vi "Telecommunications Parametric Testing.vi"() -> ()   [LabVIEW 2018]
doc: "The T1 Parametric testing application performs parametric testing of T1 signals. The T1 signal is a 1.544 Mb/s pulsed digital signal formed by multiplexing 24 voice channels. Each channel is sampled at 8000 samples/sec. Each sample is then converted to 8 bits using Pulse Coded Multiplexing. The 24 channels are then time-division multiplexed. Each frame, which corresponds to one sampling period, contains 192 bits ( 8 times 24) plus one bit for frame synchronization. Since frames occur at 8000 times per second, the bit rate is 1.544 Mb/s\n\nThis application performs the following parametric tests on T1 signals:\n\n1. Mask Test: Compares T1 signals with standard masks. The type of masks that are supported are ITU G.703 mask, EIA/TIA 547 and ANSI T1.102. The graph shows the mask in grey, the actual signal in green and failures as red squares. A boolean indicates whether the signal passed or failed the mask test and the indicator Number of Hits shows the number of times the signal did not pass the mask test.\n\n2. Measure T1 signal amplitude : Measures the amplitude of the T1 signal. The peak amplitude is displayed in the indicator Measured Amplitude.\n\n3. Measure T1 signal frequency : Measures the frequency of the T1 signal. The signal frequency in MHz is displayed in the indicator Measured Frequency."
uses:
  <vilib>/addons/database/Connection.llb/DB Tools Open Connec (Path).vi
  <vilib>/addons/database/NI_Database_API.lvlib
panel:
  in  "Stop":bool
  in  "Launch Retrieval VI":bool
  in  "Launch Logging VI":bool
  # "Overview: Demonstrates a sample application that logs data to a database and retrieves data from the database.\nRequirements: Database Connectivity Toolkit\nInstructions:\n1. Run the VI.\n2. Click Launch Logging VI to launch a VI that logs data to a database.\n3. Click Launch Retrieval VI to launch a VI that retrieves data from the database.\n4. Click Stop to stop the VI."
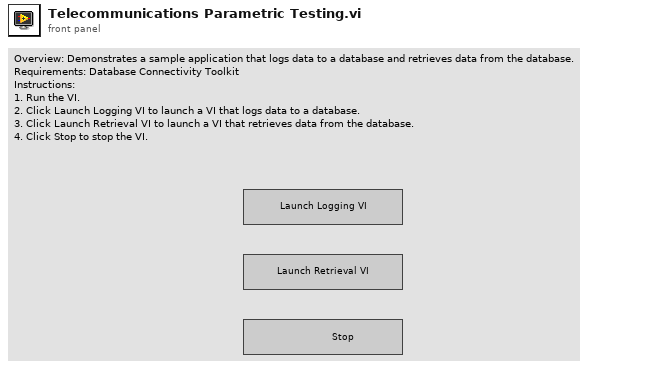
[diagram p1: front panel]
types:
  T1 = typedef "NI_Database_API.lvlib/Conn ObjectReference.ctl" = refnum<k1>
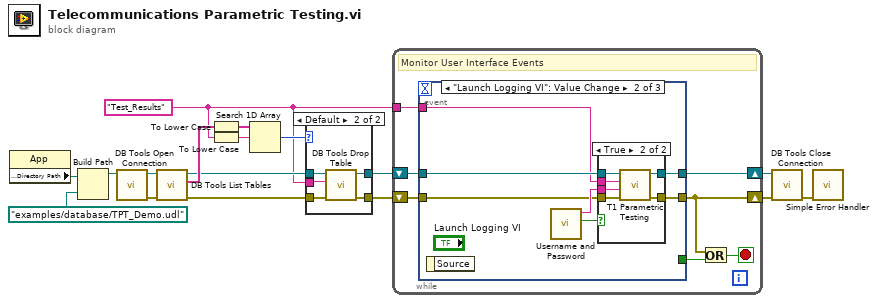
[diagram p0: block diagram]
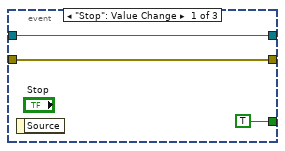
[diagram p2: hidden frame]
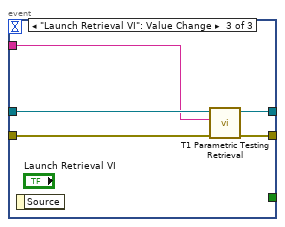
[diagram p4: hidden frame]
diagram:
  w1 = "Test_Results" ("element")
  n1 = property class="App"() -> ("Application:Directory Path"=w14:path)  [unwired: 2 in, 2 out]
  n2 = Build Path(base path=w14, name or relative path=path "examples/database/TPT_Demo.udl" ("Application:Directory Path")) -> (appended path=w12:path)
  n3 = call-poly <vilib>:"DB Tools Open Connection.vi"("connection information"=w12) -> ("error out"=w16:errorcluster, "connection reference"=w15:T1)  [unwired: 7 in]
  n4 = call <vilib>:"DB Tools List Tables.vi"("error in (no error)"=w16, "connection reference"=w15) -> ("error out"=w11:errorcluster, "tables"=w17:string[], "connection reference out"=w10:T1)  [unwired: 3 in]
  n5 = To Lower Case(string=w17) -> (all lower case string=w3:string[])
  n6 = To Lower Case(string=w1) -> (all lower case string=w2:string)
  n7 = Search 1D Array(1D array=w3, element=w2) -> (index of element=w4:i32)  [unwired: 1 in]
  n8 = case shown="Default" w4 {
    tunnel: w10 -> [w19 w23]
    tunnel: w11 -> [w18 w24]
    tunnel: [w19 w22] -> w7
    tunnel: [w18 w21] -> w8
    tunnel: w1 -> [_ w20]
    frame -1 {
    }
    frame Default {
      n9 = call <vilib>:"DB Tools Drop Table.vi"("error in (no error)"=w24, "table"=w20, "connection reference"=w23) -> ("error out"=w21:errorcluster, "connection reference out"=w22:T1)  [unwired: 5 in]
    }
  }
  n10 = while {
    shift-left: w8 -> [w30]
    shift-right: [w27] -> w5
    shift-left: w7 -> [w29]
    shift-right: [w28] -> w6
    tunnel: w1 -> [w25]
    stop <- w31 stop-if-true
    # "Monitor User Interface Events"
    n11 = event shown="[1] \"Launch Logging VI\": Value Change" {
      selector: _ -> [_ _ _]
      dyn-events: _ -> [_ _ _]
      timeout: _ -> [_ _ _]
      tunnel: w30 -> [w34 w38 w53]
      tunnel: [w34 w35 w51] -> w27
      tunnel: w29 -> [w33 w37 w54]
      tunnel: [w33 w41 w52] -> w28
      tunnel: [TRUE _ _] -> w26
      tunnel: w25 -> [_ w36 w50]
      event "Stop": Value Change {
        n12 = event-data() -> ()  [unwired: 1 in, 1 out]
      }
      event "Launch Logging VI": Value Change {
        n13 = event-data() -> ()  [unwired: 1 in, 1 out]
        n14 = call "Username and Password.vi"() -> ("Logged In?"=w39:bool, "User name out"=w40:string)  [unwired: 10 in]
        n15 = case shown="True" w39 {
          tunnel: w40 -> [_ w44]
          tunnel: w37 -> [w43 w49]
          tunnel: w38 -> [w42 w48]
          tunnel: [w43 w47] -> w41
          tunnel: [w42 w46] -> w35
          tunnel: w36 -> [_ w45]
          frame False {
          }
          frame True {
            n16 = call "T1 Parametric Testing.vi"("error in (no error)"=w48, "Operator"=w44, "table name"=w45, "connection reference"=w49) -> ("error out"=w46:errorcluster, "connection reference out"=w47:T1)  [unwired: 6 in]
          }
        }
      }
      event "Launch Retrieval VI": Value Change {
        n17 = event-data() -> ()  [unwired: 1 in, 1 out]
        n18 = call "T1 Parametric Testing Retrieval.vi"("error in (no error)"=w53, "table name"=w50, "connection reference"=w54) -> ("error out"=w51:errorcluster, "connection reference out"=w52:T1)  [unwired: 7 in]
      }
    }
    n19 = Or(x=w27, y=w26) -> (x .or. y?=w31:bool)
  }
  n20 = call <vilib>:"DB Tools Close Connection.vi"("error in (no error)"=w5, "connection reference"=w6) -> ("error out"=w9:errorcluster)  [unwired: 5 in]
  n21 = call <vilib>:"Simple Error Handler.vi"("error in (no error)"=w9) -> ()  [unwired: 4 in, 5 out]
